vi "ConfigurationSetting_Dialog.vi"(2 "error in (no error)":errorcluster, 3 "Configuration":refnum<vi>) -> (0 "error out":errorcluster, 1 "Cancelled?":bool)   [LabVIEW 2012]
doc: "Use this template to create a dialog box with event handling."
uses:
  Config.ctl
panel:
  in  "Configuration Settings":T1={"IntTime"=100, "Samples"=3, "PowerMin"=400.0, "KneeMin"=-20.0, "KneeMax"=20.0, "Background Wl"=275.0, "Settle Delay,ms"=275, "StationId"=0.0} {"Background Wl" min=220.0 max=320.0; "IntTime" min=1 max=100000; "Samples" min=1 max=10; "PowerMin" min=0.0 max=10000.0; "KneeMin" min=-40.0 max=0.0; "KneeMax" min=0.0 max=40.0}
  in  "Unblock":bool
  in  "Cancel":bool
  in  "Save":bool
  # "Measurement Settings"
  # "Test Criteria"
  # "Measurement Settings"
  # "Test Criteria"
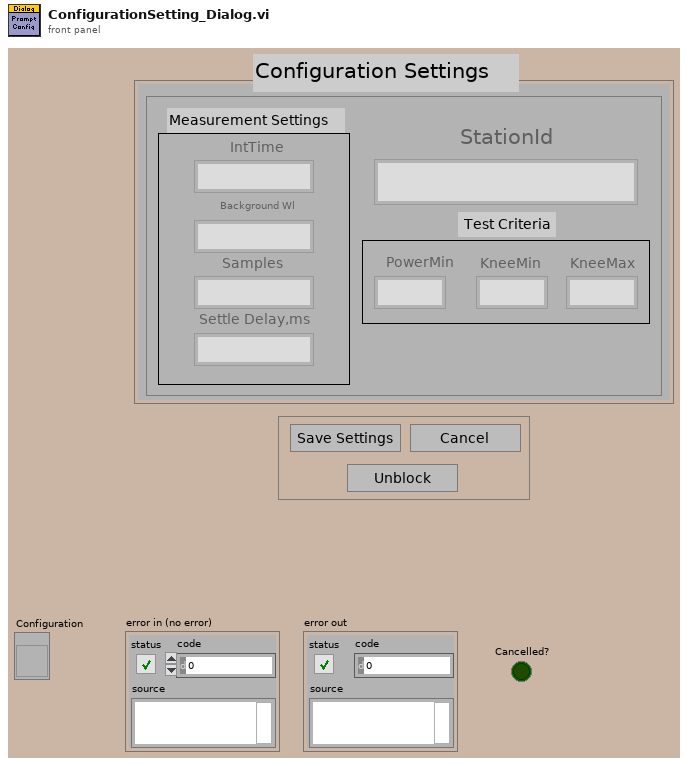
[diagram p1: front panel]
types:
  T1 = typedef "Config.ctl" = cluster{"IntTime":i32, "Samples":i32, "PowerMin":dbl, "KneeMin":dbl, "KneeMax":dbl, "Background Wl":dbl, "Settle Delay,ms":u32, "StationId":sgl}
  T2 = enum8{"Enabled", "Disabled", "Disabled and Grayed Out"}
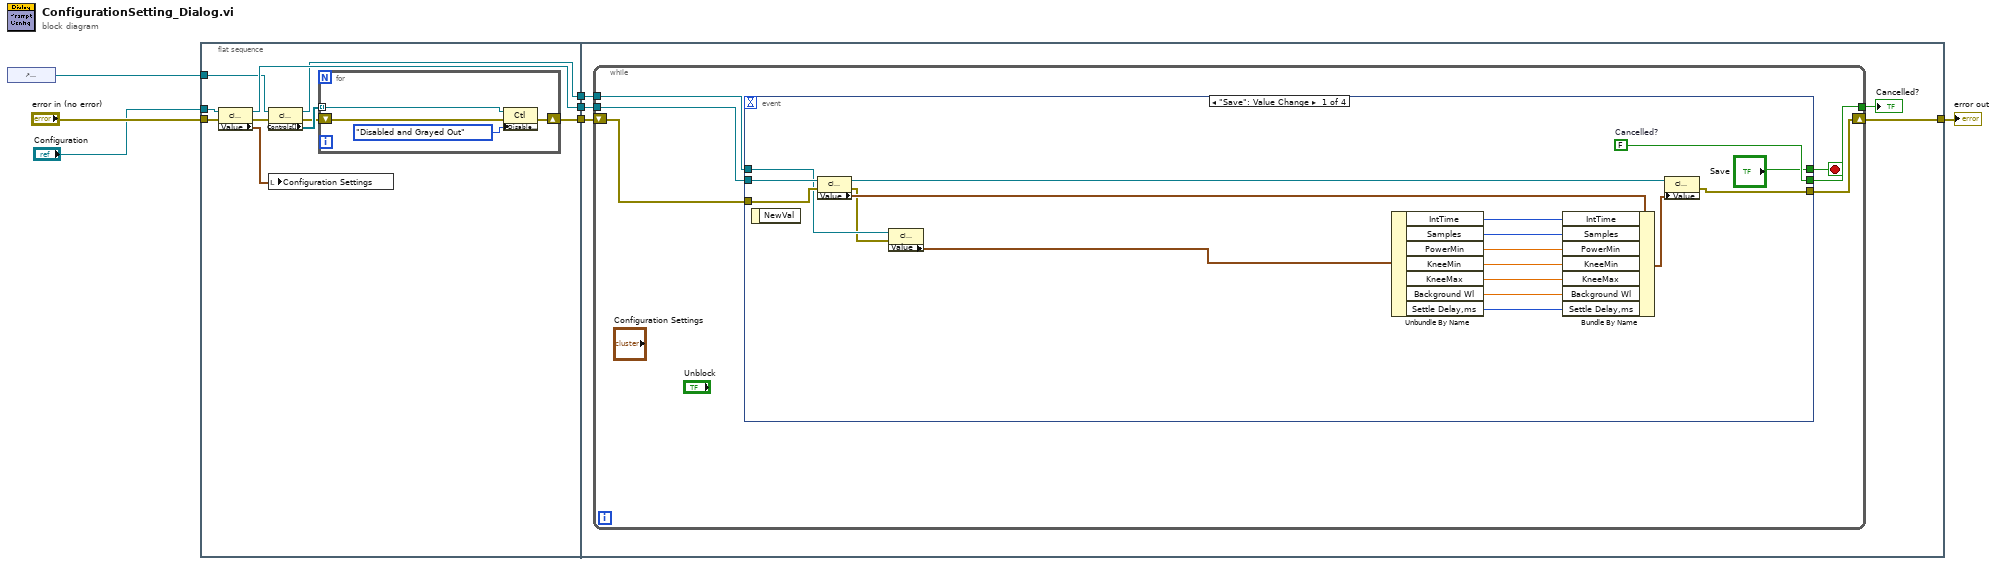
[diagram p0: block diagram]
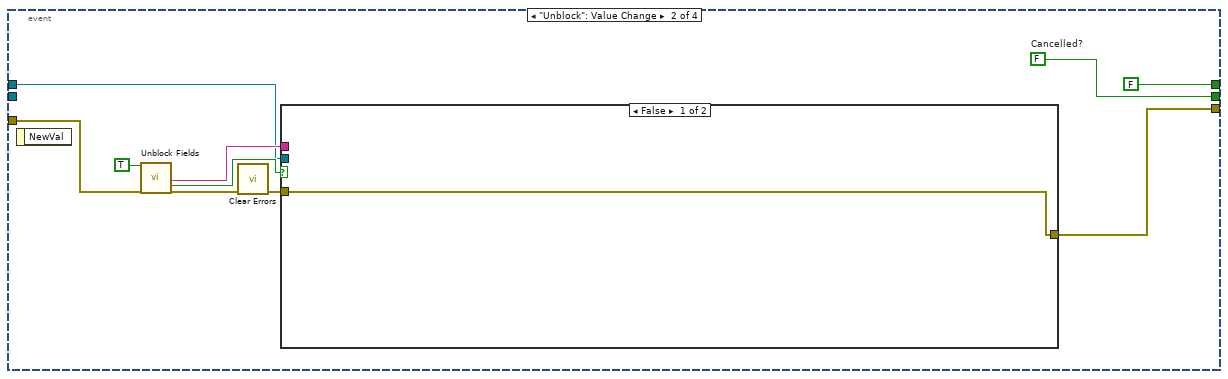
[diagram p2: hidden frame]
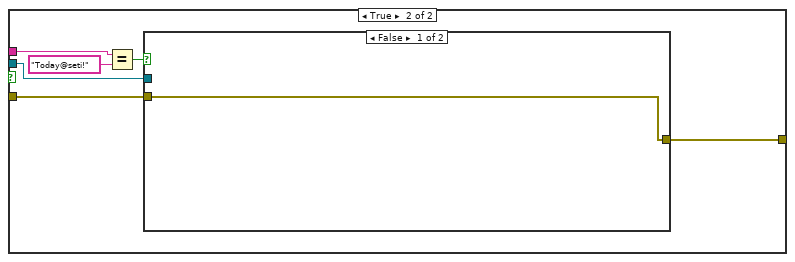
[diagram p3: hidden frame]
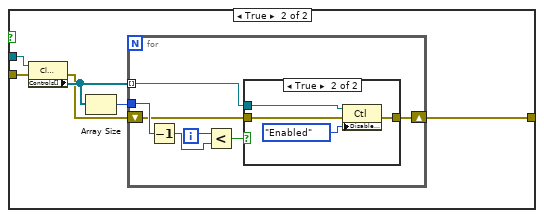
[diagram p4: hidden frame]
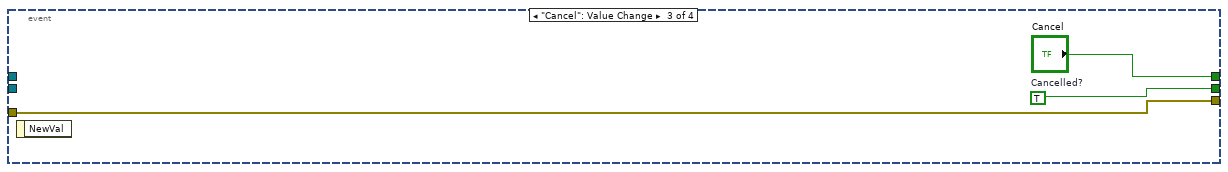
[diagram p6: hidden frame]
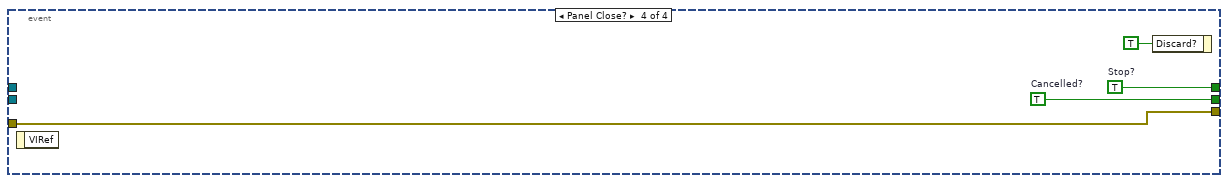
[diagram p7: hidden frame]
diagram:
  n1 = control-ref of="Configuration Settings"() -> (w3:refnum<vi>)
  n2 = flat-sequence {
    tunnel: "error in (no error)" -> [w16]
    tunnel: [w15] -> w6
    tunnel: "Configuration" -> [w17]
    tunnel: w3 -> [w12]
    tunnel: [w11] -> w2
    tunnel: [w8] -> w1
    tunnel: w6 -> [w24]
    tunnel: [w26] -> w5
    tunnel: w2 -> [w23]
    tunnel: w1 -> [w22]
    frame #0 {
      n3 = property class="Clust (strict)"(reference=w17, error in=w16) -> (reference out=w15:refnum<vi>, error out=w14:errorcluster, "Value"=w13:T1)
      n4 = property class="Clust (strict)"(reference=w12, error in=w14) -> (reference out=w11:refnum<vi>, error out=w9:errorcluster, "Controls[]"=w10:refnum<vi>[])
      n5 = local write "Configuration Settings"(w13) -> ()
      n6 = for {
        tunnel: w10 -> [w21] mode=indexing
        shift-right: [w19] -> w8
        shift-left: w9 -> [w20]
        n7 = property class="Ctl"(reference=w21, error in=w20, "DisabledEnum"=T2."Disabled and Grayed Out" ("Disabled")) -> (error out=w19:errorcluster)  [unwired: 1 out]
      }
    }
    frame #1 {
      n8 = while {
        shift-right: [w30] -> w26
        shift-left: w22 -> [w31]
        tunnel: [w29] -> w25
        tunnel: w24 -> [w28]
        tunnel: w23 -> [w27]
        stop <- w32 stop-if-true
        n9 = event shown="[0] \"Save\": Value Change" {
          selector: _ -> [_ _ _ _]
          dyn-events: _ -> [_ _ _ _]
          timeout: _ -> [_ _ _ _]
          tunnel: ["Save" FALSE ("Stop?") "Cancel" w92] -> w32
          tunnel: [w50 w60 w89 w91] -> w29
          tunnel: w31 -> [w47 w58 w87 w90]
          tunnel: [w45 w54 w87 w90] -> w30
          tunnel: w28 -> [w48 _ _ _]
          tunnel: w27 -> [w35 w51 _ _]
          event "Save": Value Change {
            w50 = FALSE  # Cancelled?
            n10 = event-data() -> ()  [unwired: 1 in, 1 out]
            n11 = property class="Clust (strict)"(reference=w48, error in=w47) -> (reference out=w46:refnum<vi>, error out=w34:errorcluster, "Value"=w44:T1)
            n12 = property class="Clust (strict)"(reference=w35, error in=w34) -> ("Value"=w33:T1)  [unwired: 2 out]
            n13 = Unbundle By Name(w33) -> ("IntTime"=w43:i32, "Samples"=w42:i32, "PowerMin"=w41:dbl, "KneeMin"=w40:dbl, "KneeMax"=w39:dbl, "Background Wl"=w38:dbl, "Settle Delay,ms"=w37:u32)
            n14 = Bundle By Name(cluster=w44, "IntTime"=w43, "Samples"=w42, "PowerMin"=w41, "KneeMin"=w40, "KneeMax"=w39, "Background Wl"=w38, "Settle Delay,ms"=w37) -> (w36:T1)
            n15 = property class="Clust (strict)"(reference=w46, "Value"=w36) -> (error out=w45:errorcluster)  [unwired: 1 in, 1 out]
          }
          event "Unblock": Value Change {
            w60 = FALSE  # Cancelled?
            n16 = event-data() -> ()  [unwired: 1 in, 1 out]
            n17 = call "Unblock Fields"("Enable"=TRUE, "error in (no error)"=w58) -> ("Password"=w52:string, "OK"=w56:bool, "error out"=w57:errorcluster)  [unwired: 15 in]
            n18 = call <vilib>:"Clear Errors.vi"("error in (no error)"=w57) -> ("error out"=w55:errorcluster)  [unwired: 6 in]
            n19 = case shown="False" w56 {
              tunnel: w55 -> [w61 w63]
              tunnel: [w61 w64] -> w54
              tunnel: w52 -> [_ w67]
              tunnel: w51 -> [_ w62]
              frame False {
              }
              frame True {
                n20 = Equal?(x=w67, y="Today@seti!") -> (x = y?=w65:bool)
                n21 = case shown="False" w65 {
                  tunnel: [w68 w69] -> w64
                  tunnel: w63 -> [w68 w72]
                  tunnel: w62 -> [_ w73]
                  frame False {
                  }
                  frame True {
                    n22 = property class="Clust (strict)"(reference=w73, error in=w72) -> (error out=w70:errorcluster, "Controls[]"=w71:refnum<vi>[])  [unwired: 1 out]
                    n23 = Array Size(array=w71) -> (size(s)=w74:i32)
                    n24 = for {
                      tunnel: w71 -> [w81] mode=indexing
                      tunnel: w74 -> [w80]
                      shift-right: [w77] -> w69
                      shift-left: w70 -> [w78]
                      i -> [w76]
                      n25 = Decrement(x=w80) -> (x-1=w75:i32)
                      n26 = Less?(x=w76, y=w75) -> (x < y?=w79:bool)
                      n27 = case shown="True" w79 {
                        tunnel: w81 -> [_ w86]
                        tunnel: w78 -> [w82 w84]
                        tunnel: [w82 w83] -> w77
                        frame False {
                        }
                        frame True {
                          n28 = property class="Ctl"(reference=w86, error in=w84, "DisabledEnum"=T2."Enabled" ("Disabled")) -> (error out=w83:errorcluster)  [unwired: 1 out]
                        }
                      }
                    }
                  }
                }
              }
            }
          }
          event "Cancel": Value Change {
            w89 = TRUE  # Cancelled?
            n29 = event-data() -> ()  [unwired: 1 in, 1 out]
          }
          event Panel Close? {
            w91 = TRUE  # Cancelled?
            w92 = TRUE  # Stop?
            n30 = event-data() -> ()  [unwired: 1 in, 1 out]
            n31 = event-data("Discard?"=TRUE) -> ()  [unwired: 1 in, 1 out]
          }
        }
      }
      "Cancelled?" <- w25
    }
  }
  "error out" <- w5
